vi "wola_4.vi"(9 "input valid":bool, 10 "data in":u32) -> (0 "new fft loop":bool, 1 "output valid":bool, 2 "Q":fxp<+/-,21,18>, 3 "I":fxp<+/-,21,18>)   [LabVIEW 2021]
uses:
  <vilib>/rvi/Memory/Memory_Emulation/nirvimemoryFastEmulation.vi
  <vilib>/rvi/Memory/Memory_Emulation/nirvimemoryEmulation.vi
  <vilib>/rvi/Emulation/niFpgaEmulationIsFPGAContextNoSignature.vi
  <vilib>/rvi/DataTransferAndStorage/Container/Common/niFpgaContainerGetUniqueNameForEmu.vi
  <vilib>/rvi/Emulation/niFpgaProcessEmulError.vi
  <vilib>/rvi/Emulation/niFpgaSctlEmulationGetInTimedLoop.vi
  <vilib>/rvi/errors/nirviReportUnexpectedCaseInternalError (U32).vi
  <vilib>/rvi/FXPMathLib/FxpAdd/XNode/nifxpmath_Add.xnode
  <vilib>/rvi/DataTransferAndStorage/Container/XNode/niFpgaContainer.xnode
  <vilib>/rvi/FXPMathLib/sim/FxpSim.dll
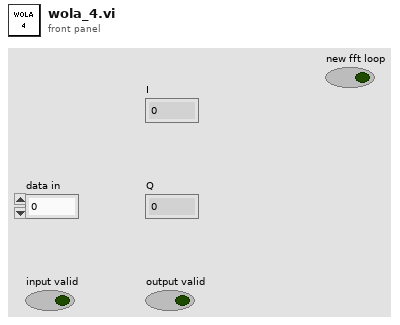
[diagram p1: front panel]
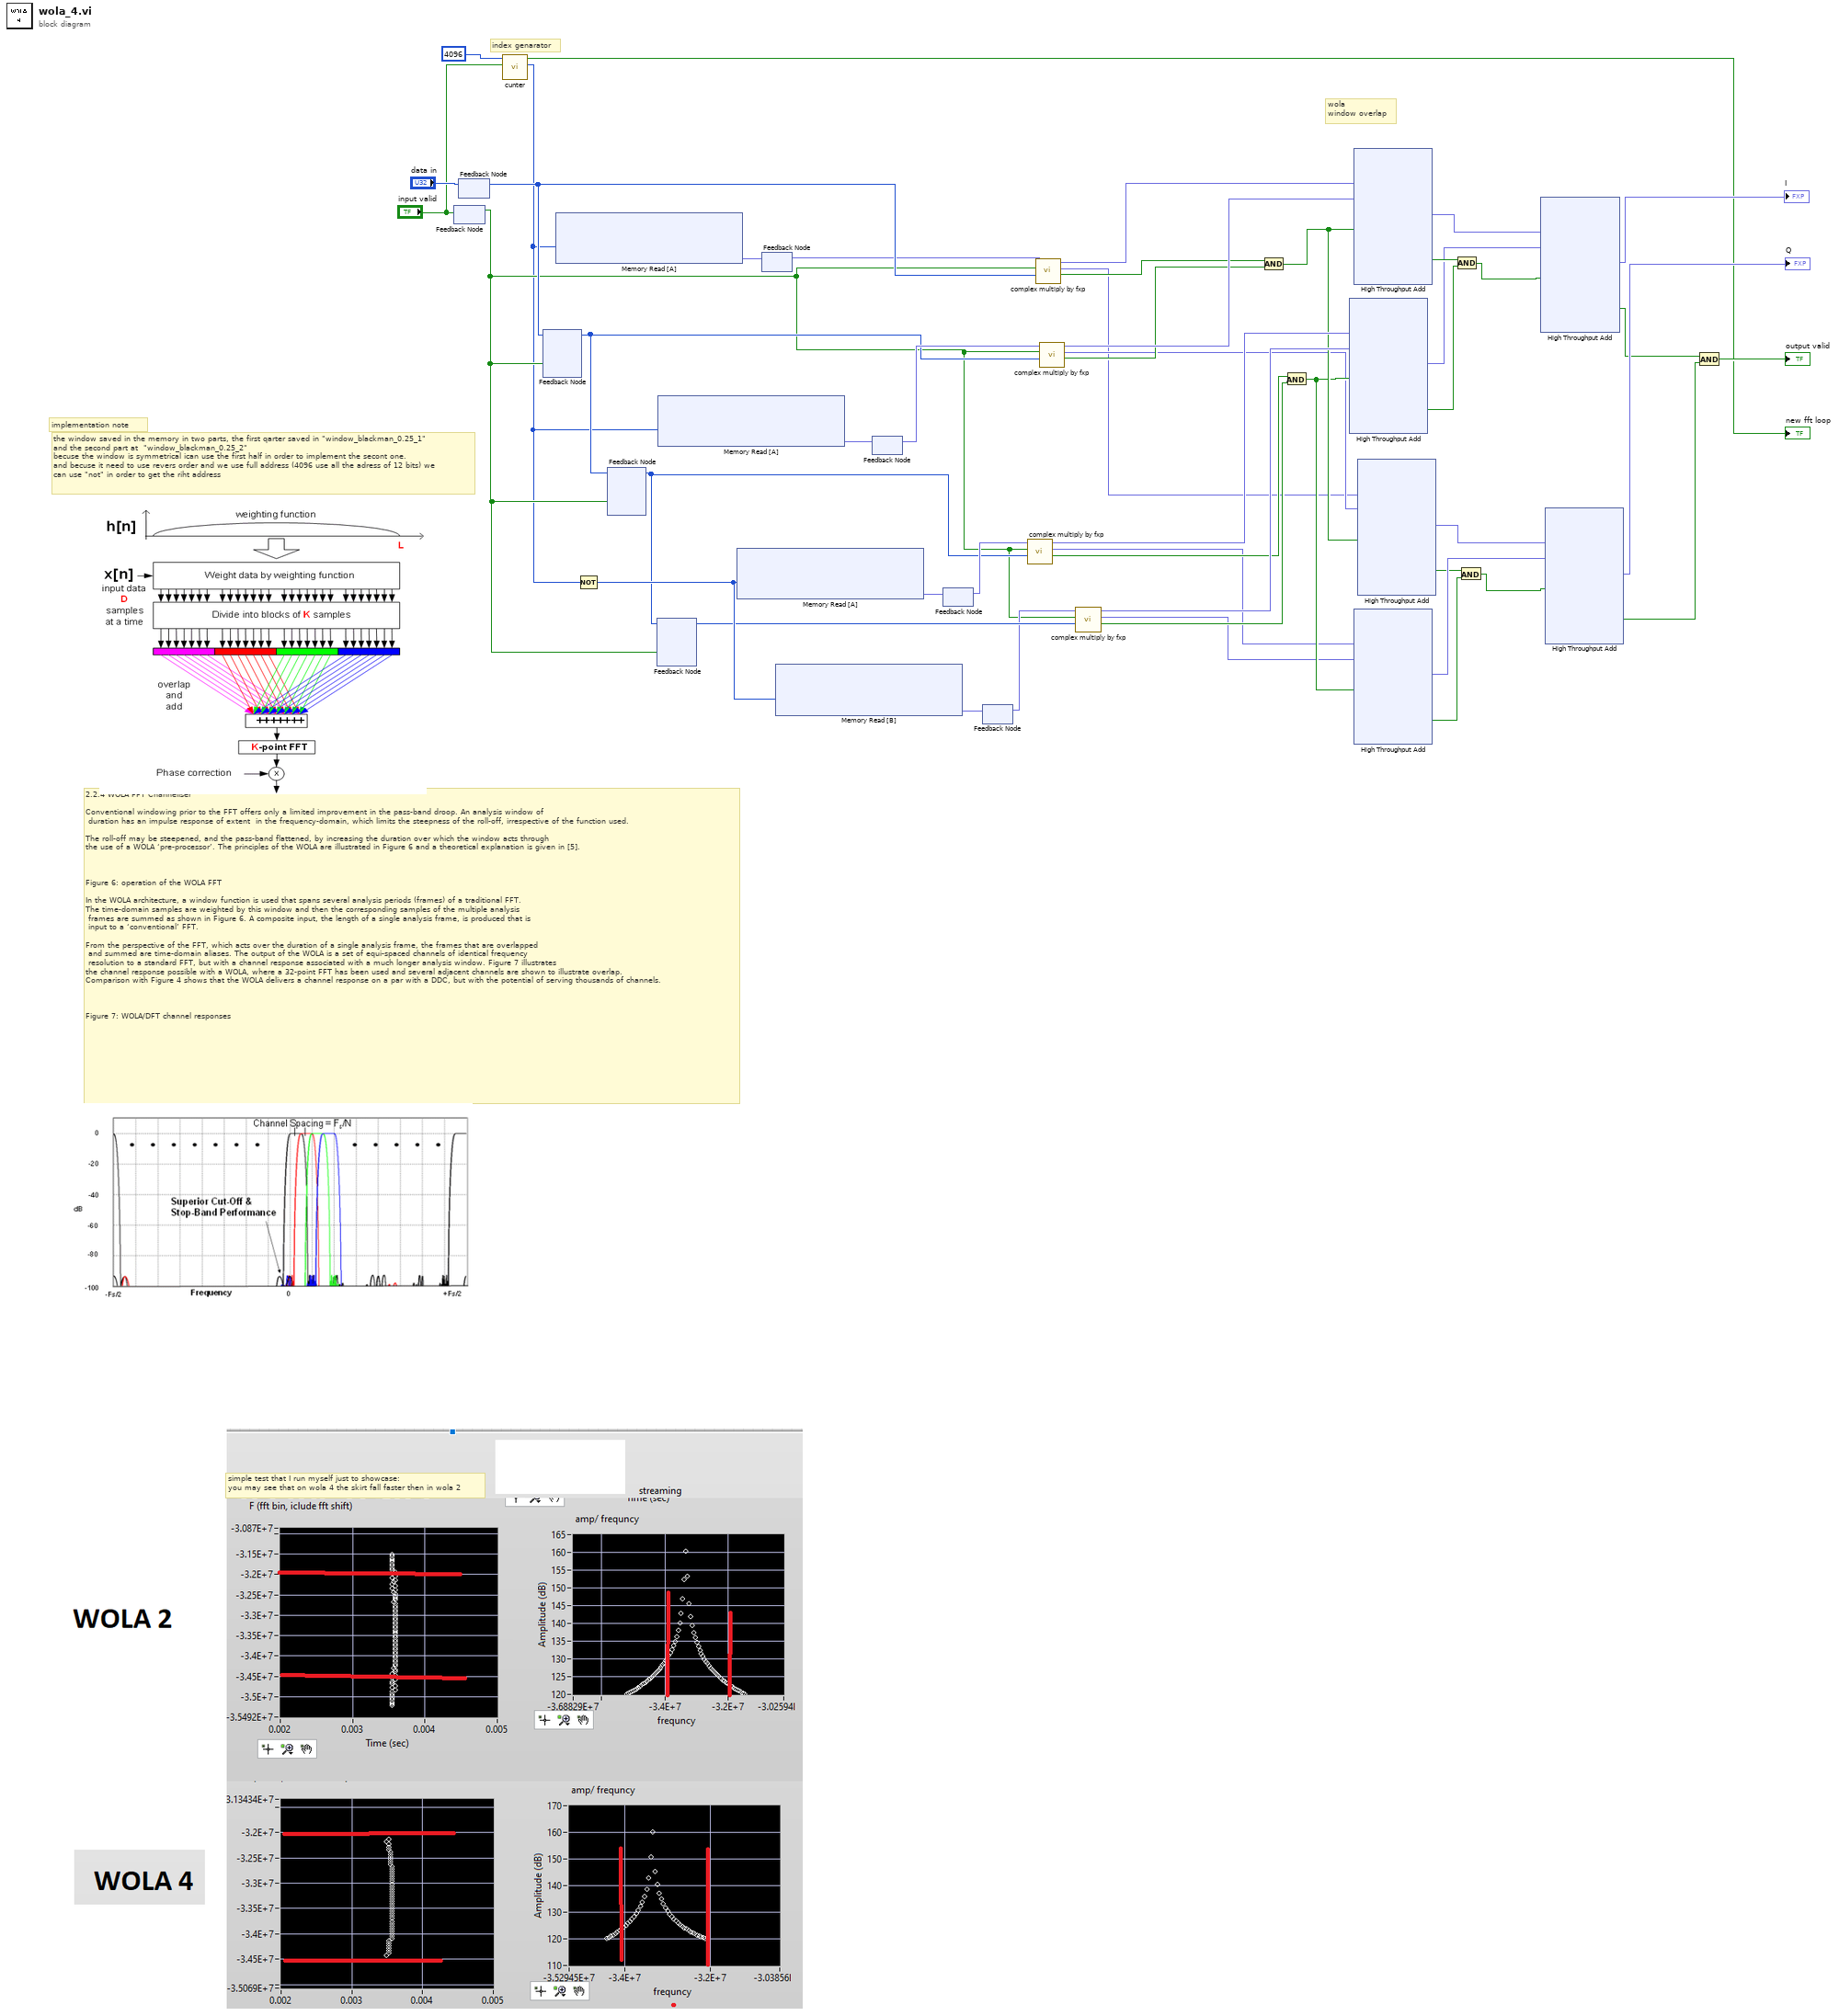
[diagram p0: block diagram]
diagram:
  # "implementation note"
  # "simple test that I run myself just to showcase:\nyou may see that on wola 4 the skirt fall faster then in wola 2"
  # "2.2.4 WOLA FFT Channeliser\n\nConventional windowing prior to the FFT offers only a limited improvement in the pass-band droop. An analysis window of\n duration has an impulse response of extent  in the frequency-domain, which limits the steepness of the roll-off, irrespective of the function used.\n\nThe roll-off may be steepened, and the pass-band flattened, by increasing the duration over which the window acts through \nthe use of a WOLA ‘pre-processor’. The principles of the WOLA are illustrated in Figure 6 and a theoretical explanation is given in [5].\n\n\n\nFigure 6: operation of the WOLA FFT\n\nIn the WOLA architecture, a window function is used that spans several analysis periods (frames) of a traditional FFT. \nThe time-domain samples are weighted by this window and then the corresponding samples of the multiple analysis\n frames are summed as shown in Figure 6. A composite input, the length of a single analysis frame, is produced that is\n input to a ‘conventional’ FFT.\n\nFrom the perspective of the FFT, which acts over the duration of a single analysis frame, the frames that are overlapped\n and summed are time-domain aliases. The output of the WOLA is a set of equi-spaced channels of identical frequency\n resolution to a standard FFT, but with a channel response associated with a much longer analysis window. Figure 7 illustrates \nthe channel response possible with a WOLA, where a 32-point FFT has been used and several adjacent channels are shown to illustrate overlap. \nComparison with Figure 4 shows that the WOLA delivers a channel response on a par with a DDC, but with the potential of serving thousands of channels.\n\n\n\nFigure 7: WOLA/DFT channel responses"
  # "the window saved in the memory in two parts, the first qarter saved in \"window_blackman_0.25_1\" \nand the second part at  \"window_blackman_0.25_2\"\nbecuse the window is symmetrical ican use the first half in order to implement the secont one.\nand becuse it need to use revers order and we use full address (4096 use all the adress of 12 bits) we\ncan use \"not\" in order to get the riht address"
  # "index genarator"
  # "wola\nwindow overlap"
  n1 = feedback #1() -> (w5:bool)  [unwired: 1 in]
  n2 = feedback-in #1("input valid") -> ()
  n3 = feedback #2() -> (w44:u32)  [unwired: 1 in]
  n4 = feedback-in #2("data in") -> ()
  n5 = call "cunter.vi"("input valid"="input valid", "count to"=u16 4096 ("x")) -> ("count"=w2:u16, "reset (out)"=→"new fft loop":bool)  [unwired: 8 in]
  n6 = feedback #3() -> (w37:u32)  [unwired: 1 in]
  n7 = feedback-in #3(w44, w5) -> ()
  n8 = xnode ("Memory Read [A]")("Address A"=w2) -> ("Data A"=w46:fxp<+,16,0>)  [unwired: 1 in, 1 out]
  n9 = Not(x=w2) -> (.not. x?=w39:u16)
  n10 = feedback #4() -> (w33:u32)  [unwired: 1 in]
  n11 = feedback-in #4(w37, w5) -> ()
  n12 = feedback #5() -> (w35:u32)  [unwired: 1 in]
  n13 = feedback-in #5(w33, w5) -> ()
  n14 = xnode ("Memory Read [A]")("Address B"=w2) -> ("Data B"=w42:fxp<+,16,0>)  [unwired: 1 in, 1 out]
  n15 = xnode ("Memory Read [A]")("Address A"=w39) -> ("Data A"=w40:fxp<+,16,0>)  [unwired: 1 in, 1 out]
  n16 = feedback-in #6(w46) -> ()
  n17 = feedback #6() -> (w43:fxp<+,16,0>)  [unwired: 1 in]
  n18 = xnode ("Memory Read [B]")("Address B"=w39) -> ("Data B"=w38:fxp<+,16,0>)  [unwired: 1 in, 1 out]
  n19 = feedback #7() -> (w41:fxp<+,16,0>)  [unwired: 1 in]
  n20 = feedback-in #7(w42) -> ()
  n21 = feedback #8() -> (w36:fxp<+,16,0>)  [unwired: 1 in]
  n22 = feedback-in #8(w40) -> ()
  n23 = feedback #9() -> (w34:fxp<+,16,0>)  [unwired: 1 in]
  n24 = feedback-in #9(w38) -> ()
  n25 = call "complex multiply by fxp.vi"("data in"=w33, "input valid"=w5, "Data A"=w36) -> ("data valid"=w23:bool, "Q"=w13:fxp<+/-,19,16>, "I"=w30:fxp<+/-,19,16>)  [unwired: 6 in]
  n26 = call "complex multiply by fxp.vi"("data in"=w44, "input valid"=w5, "Data A"=w43) -> ("data valid"=w25:bool, "Q"=w11:fxp<+/-,19,16>, "I"=w32:fxp<+/-,19,16>)  [unwired: 6 in]
  n27 = call "complex multiply by fxp.vi"("data in"=w37, "input valid"=w5, "Data A"=w41) -> ("data valid"=w24:bool, "Q"=w12:fxp<+/-,19,16>, "I"=w31:fxp<+/-,19,16>)  [unwired: 6 in]
  n28 = call "complex multiply by fxp.vi"("data in"=w35, "input valid"=w5, "Data A"=w34) -> ("data valid"=w22:bool, "Q"=w14:fxp<+/-,19,16>, "I"=w29:fxp<+/-,19,16>)  [unwired: 6 in]
  n29 = And(x=w25, y=w24) -> (x .and. y?=w16:bool)
  n30 = And(x=w23, y=w22) -> (x .and. y?=w15:bool)
  n31 = xnode ("High Throughput Add")("x"=w30, "y"=w29, "input valid"=w15) -> ("x+y"=w27:fxp<+/-,20,17>, "output valid"=w48:bool)  [unwired: 1 in, 1 out]
  n32 = xnode ("High Throughput Add")("x"=w32, "y"=w31, "input valid"=w16) -> ("x+y"=w28:fxp<+/-,20,17>, "output valid"=w47:bool)  [unwired: 1 in, 1 out]
  n33 = xnode ("High Throughput Add")("x"=w13, "y"=w14, "input valid"=w15) -> ("x+y"=w20:fxp<+/-,20,17>, "output valid"=w17:bool)  [unwired: 1 in, 1 out]
  n34 = xnode ("High Throughput Add")("x"=w11, "y"=w12, "input valid"=w16) -> ("x+y"=w19:fxp<+/-,20,17>, "output valid"=w18:bool)  [unwired: 1 in, 1 out]
  n35 = And(x=w47, y=w48) -> (x .and. y?=w26:bool)
  n36 = And(x=w18, y=w17) -> (x .and. y?=w21:bool)
  n37 = xnode ("High Throughput Add")("x"=w28, "y"=w27, "input valid"=w26) -> ("x+y"=→"I":fxp<+/-,21,18>, "output valid"=w8:bool)  [unwired: 1 in, 1 out]
  n38 = xnode ("High Throughput Add")("x"=w19, "y"=w20, "input valid"=w21) -> ("x+y"=→"Q":fxp<+/-,21,18>, "output valid"=w7:bool)  [unwired: 1 in, 1 out]
  n39 = And(x=w8, y=w7) -> (x .and. y?=→"output valid":bool)
